vi "DDMs_low_measure.vi"(7 "Sample #":i32=5, 8 "error in (no error)":errorcluster, 9 "Measurement":T1(ring), 10 "Device":T2(ring), 11 "VISA resource name":refnum<visa-resource-name>) -> (0 "error out":errorcluster, 2 "Measurement":dbl format="%0.2f", 3 "VISA resource name out":refnum<visa-resource-name>)   [LabVIEW 2017, in "DMMsData.lvclass"]
uses:
  DMMsData.lvclass
  <vilib>/Analysis/baseanly.llb/Mean (DBL).vi
  <instrlib>/Agilent 34401/Public/Data/Read (Multiple Points).vi
  <instrlib>/Agilent 34401/Agilent 34401.lvlib
  <vilib>/Analysis/NI_AALBase.lvlib
  istr.lib/ADCMT7351_ADC/ADCMT7351_ADC.lvlib
  istr.lib/ADCMT7451A_ADC/ADCMT7451_ADC.lvlib
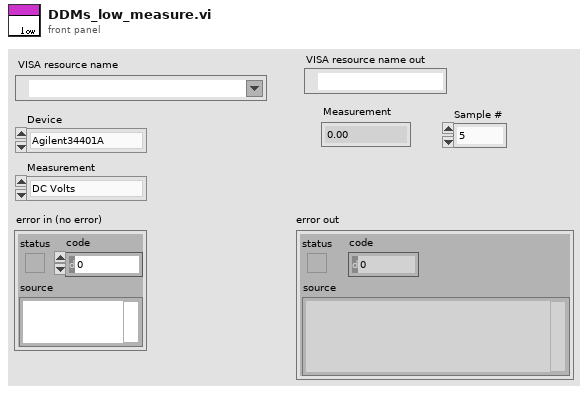
[diagram p1: front panel]
types:
  T1 = enum16{"DC Volts", "DC Currents", "2-Wire Resistance", "4-Wire Resistance"}
  T2 = enum16{"Agilent34401A", "ADCMT7351", "HP3478A", "ADCMT7451"}
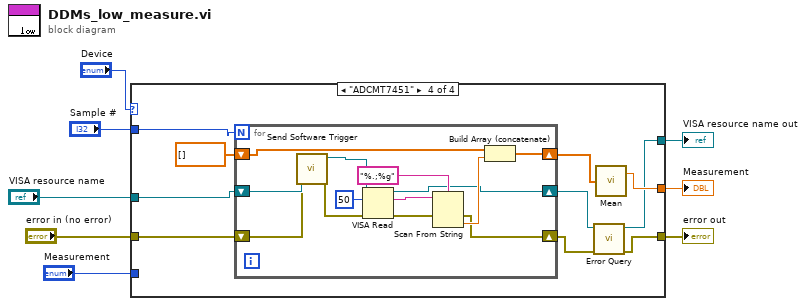
[diagram p0: block diagram]
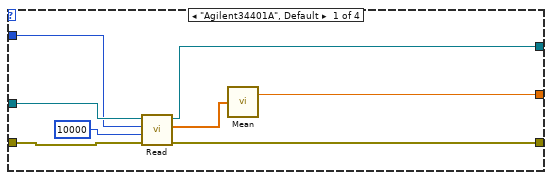
[diagram p2: hidden frame]
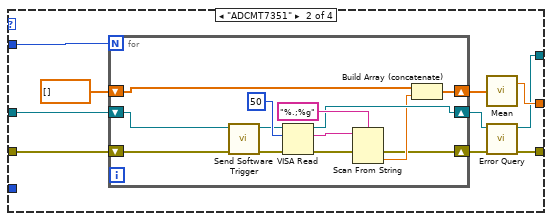
[diagram p3: hidden frame]
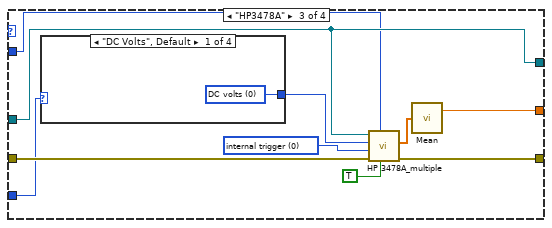
[diagram p4: hidden frame]
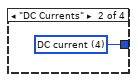
[diagram p5: hidden frame]
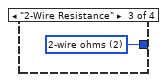
[diagram p6: hidden frame]
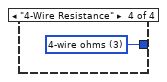
[diagram p7: hidden frame]
diagram:
  n1 = case shown="\"ADCMT7451\"" "Device" {
    tunnel: "VISA resource name" -> [w16 w24 w49 w62]
    tunnel: "error in (no error)" -> [w15 w23 w47 w61]
    tunnel: [w14 w18 w49 w54] -> w5
    tunnel: [w13 w17 w48 w56] -> w4
    tunnel: [w10 w21 w46 w58] -> w3
    tunnel: "Sample #" -> [w9 w19 w41 w63]
    tunnel: "Measurement" -> [_ _ w43 _]
    frame "Agilent34401A", Default {
      n2 = call-poly <instrlib>:"Read.vi"("error in (no error)"=w15, "Maximum Time (10000 ms)"=u32 10000, "Sample Count (1)"=w9, "VISA resource name"=w16) -> ("error out"=w13:errorcluster, "Measurements"=w11:dbl[], "VISA resource name out"=w14:refnum<visa-resource-name>)  [unwired: 5 in]
      n3 = call-poly <vilib>:"Mean.vi"("X"=w11) -> ("mean"=w10:dbl)  [unwired: 1 out]
    }
    frame "ADCMT7351" {
      n4 = for {
        N: w19 -> [_]
        shift-right: [w38] -> w22
        shift-left: dbl[] [] -> [w39]
        shift-right: [w33] -> w26
        shift-left: w24 -> [w29]
        shift-right: [w27] -> w20
        shift-left: w23 -> [w37]
        n5 = call "Send Software Trigger.vi"("error in (no error)"=w37, "VISA resource name"=w29) -> ("error out"=w32:errorcluster, "VISA resource name out"=w34:refnum<visa-resource-name>)  [unwired: 8 in]
        n6 = VISA Read(VISA resource name=w34, byte count=50, error in (no error)=w32) -> (VISA resource name out=w33:refnum<visa-resource-name>, read buffer=w31:string, error out=w28:errorcluster)  [unwired: 1 out]
        n7 = Scan From String(format string="%.;%g", input string=w31, error in=w28) -> (error out=w27:errorcluster, output 1=w30:dbl)  [unwired: 2 in, 2 out]
        n8 = Build Array (concatenate)(w39, w30) -> (w38:dbl[])
      }
      n9 = call-poly <vilib>:"Mean.vi"("X"=w22) -> ("mean"=w21:dbl)  [unwired: 1 out]
      n10 = call "Error Query.vi"("error in (no error)"=w20, "VISA resource name"=w26) -> ("error out"=w17:errorcluster, "VISA resource name out"=w18:refnum<visa-resource-name>)  [unwired: 6 in, 2 out]
    }
    frame "HP3478A" {
      w44 = i16 0 items=["internal trigger", "single trigger", "external trigger", "trigger hold", "fast trigger"] ("trigger mode")
      n11 = case shown="\"DC Volts\", Default" w43 {
        tunnel: [w50 w51 w52 w53] -> w42
        frame "DC Volts", Default {
          w50 = i16 0 items=["DC volts", "AC volts", "2-wire ohms", "4-wire ohms", "DC current", "AC current", "extended ohms"] ("measurement")
        }
        frame "DC Currents" {
          w51 = i16 4 items=["DC volts", "AC volts", "2-wire ohms", "4-wire ohms", "DC current", "AC current", "extended ohms"] ("measurement")
        }
        frame "2-Wire Resistance" {
          w52 = i16 2 items=["DC volts", "AC volts", "2-wire ohms", "4-wire ohms", "DC current", "AC current", "extended ohms"] ("measurement")
        }
        frame "4-Wire Resistance" {
          w53 = i16 3 items=["DC volts", "AC volts", "2-wire ohms", "4-wire ohms", "DC current", "AC current", "extended ohms"] ("measurement")
        }
      }
      n12 = call "HP 3478A_multiple.vi"("autorange"=TRUE, "Sample #"=w41, "error in"=w47, "trigger mode"=w44, "measurement"=w42, "VISA resource name"=w49) -> ("error out"=w48:errorcluster, "Measurements"=w40:dbl[])  [unwired: 3 in]
      n13 = call-poly <vilib>:"Mean.vi"("X"=w40) -> ("mean"=w46:dbl)  [unwired: 1 out]
    }
    frame "ADCMT7451" {
      n14 = for {
        N: w63 -> [_]
        shift-right: [w64] -> w55
        shift-left: w62 -> [w76]
        shift-right: [w67] -> w57
        shift-left: w61 -> [w71]
        shift-right: [w69] -> w59
        shift-left: dbl[] [] -> [w68]
        n15 = call "Send Software Trigger.vi"("error in (no error)"=w71, "VISA resource name"=w76) -> ("error out"=w66:errorcluster, "VISA resource name out"=w65:refnum<visa-resource-name>)  [unwired: 8 in]
        n16 = VISA Read(VISA resource name=w65, byte count=u32 50, error in (no error)=w66) -> (VISA resource name out=w64:refnum<visa-resource-name>, read buffer=w74:string, error out=w75:errorcluster)  [unwired: 1 out]
        n17 = Scan From String(format string="%.;%g", input string=w74, error in=w75) -> (error out=w67:errorcluster, output 1=w70:dbl)  [unwired: 2 in, 2 out]
        n18 = Build Array (concatenate)(w68, w70) -> (w69:dbl[])
      }
      n19 = call "Error Query.vi"("error in (no error)"=w57, "VISA resource name"=w55) -> ("error out"=w56:errorcluster, "VISA resource name out"=w54:refnum<visa-resource-name>)  [unwired: 6 in, 2 out]
      n20 = call-poly <vilib>:"Mean.vi"("X"=w59) -> ("mean"=w58:dbl)  [unwired: 1 out]
    }
  }
  "VISA resource name out" <- w5
  "error out" <- w4
  "Measurement" <- w3
